vi "populate without intermediate class.vi"() -> ()   [LabVIEW 2018]
uses:
  demo/Implementations/Component-A.lvclass
  U:/modules/labview-orm/_Serializable Base Object/_ISerializable.lvclass
  U:/modules/labview-orm/demo/Component.lvclass
  demo/Implementations/Product-A.lvclass
  U:/modules/labview-orm/demo/Product.lvclass
panel:
  out "owner":string
  out "numeric":i64
  out "serian-num":dbl
  out "mayExplode_":bool
  out "status":u8
  out "isObsolete":bool
  out "id":i32
  out "error out":errorcluster
  in  "error in (no error)":errorcluster
  out "xml string":string
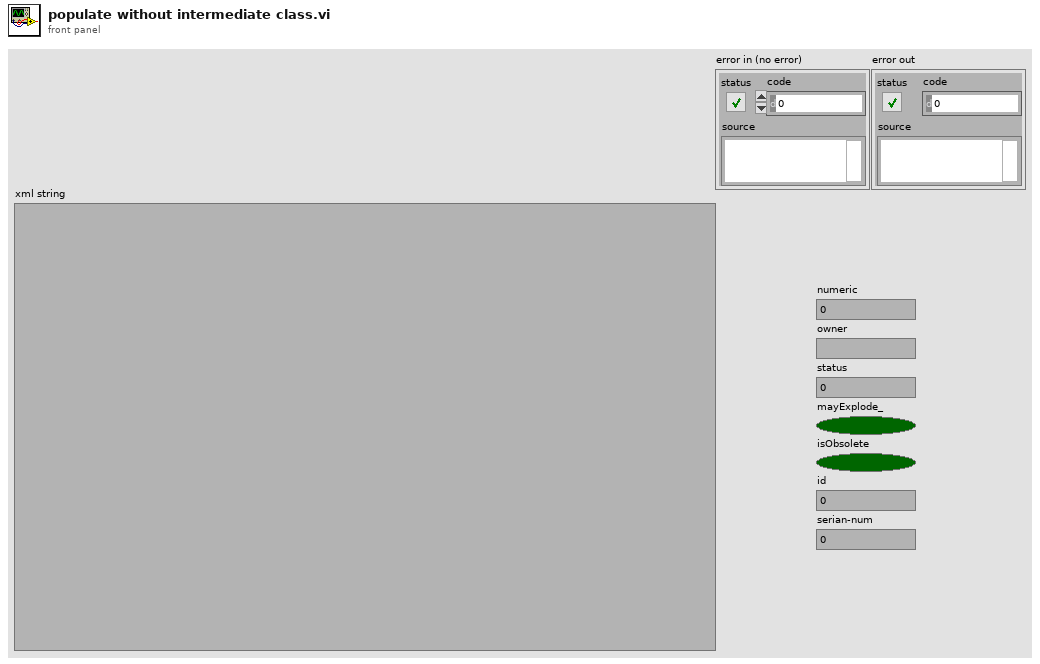
[diagram p1: front panel]
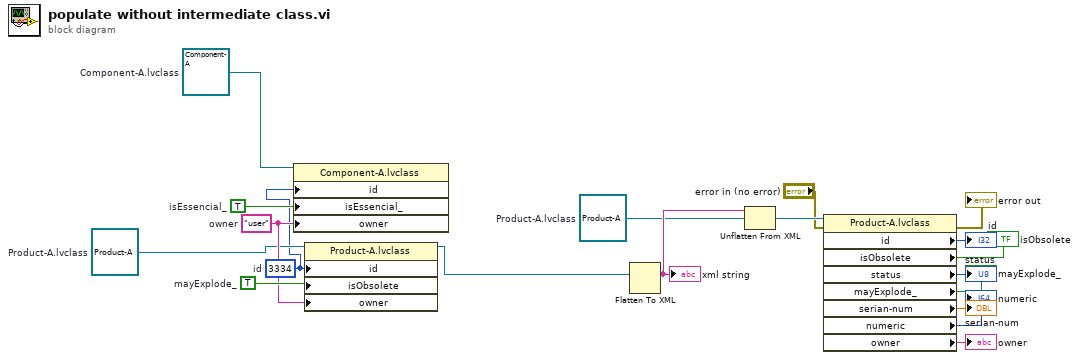
[diagram p0: block diagram]
diagram:
  w11 = refnum<class "Product-A.lvclass"> refnum  # Product-A.lvclass
  w15 = refnum<class "Product-A.lvclass"> refnum  # Product-A.lvclass
  w18 = TRUE  # mayExplode_
  w14 = 3334  # id
  w17 = "user"  # owner
  w19 = TRUE  # isEssencial_
  w16 = refnum<class "Component-A.lvclass"> refnum  # Component-A.lvclass
  n1 = property class="Component-A.lvclass"(reference=w16, "id"=w14, "isEssencial_"=w19, "owner"=w17) -> ()  [unwired: 1 in, 2 out]
  n2 = property class="Product-A.lvclass"(reference=w15, "id"=w14, "isObsolete"=w18, "owner"=w17) -> (reference out=w13:refnum<class "Product-A.lvclass">)  [unwired: 1 in, 1 out]
  n3 = Flatten To XML(anything=w13) -> (xml string=w12:string)
  "xml string" <- w12
  n4 = Unflatten From XML(xml string=w12, type=w11) -> (value=w10:refnum<class "Product-A.lvclass">)  [unwired: 1 in, 1 out]
  n5 = property class="Product-A.lvclass"(reference=w10, error in="error in (no error)") -> (error out=→"error out":errorcluster, "id"=→"id":i32, "isObsolete"=→"isObsolete":bool, "status"=→"status":u8, "mayExplode_"=→"mayExplode_":bool, "serian-num"=→"serian-num":dbl, "numeric"=→"numeric":i64, "owner"=→"owner":string)  [unwired: 1 out]
